vi "Fetch the IO Controls.vi"(0 "VI Path":path, 11 "error in (no error)":errorcluster) -> (4 "IO Controls[]":string[](array[string]), 15 "error out":errorcluster)   [LabVIEW 2021, in "Converter.lvlib"]
uses:
  Converter.lvlib
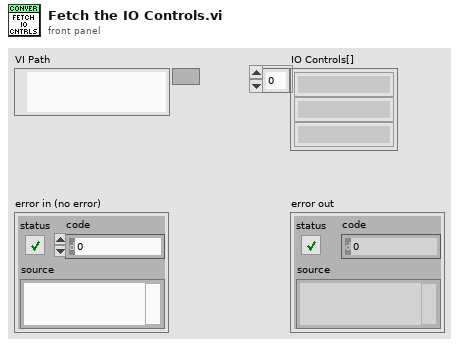
[diagram p1: front panel]
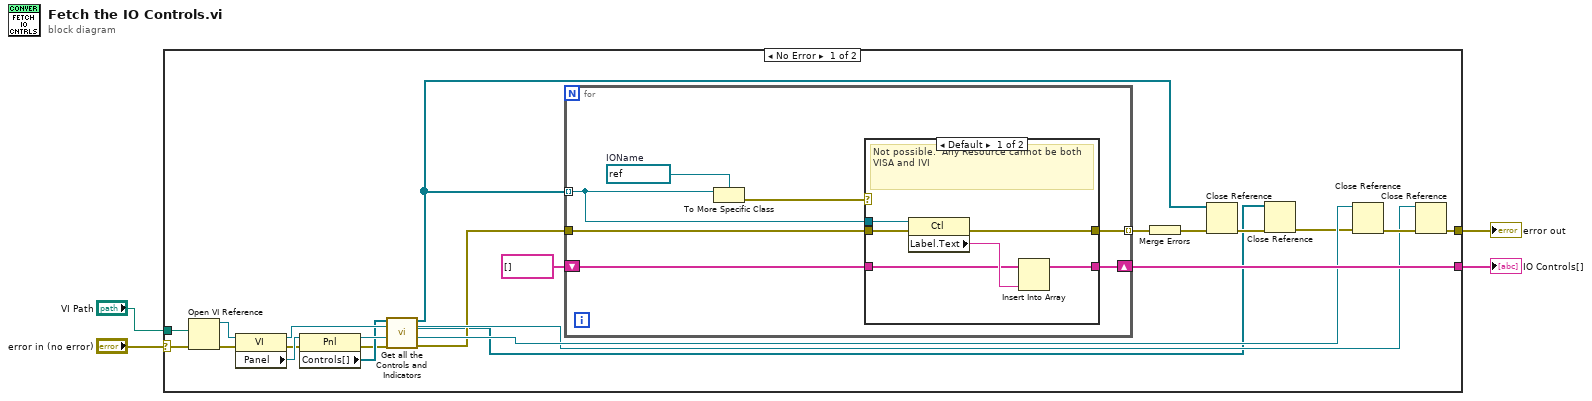
[diagram p0: block diagram]
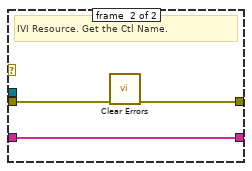
[diagram p2: hidden frame]
diagram:
  n1 = case shown="No Error" "error in (no error)" {
    selector: "error in (no error)" -> [w14 w42]
    tunnel: [w18 _] -> w4
    tunnel: [w13 w42] -> w2
    tunnel: "VI Path" -> [w12 _]
    frame No Error {
      n2 = Open VI Reference(vi path=w12, error in (no error)=w14) -> (vi reference=w25:refnum<vi>, error out=w23:errorcluster)  [unwired: 4 in]
      n3 = property class="VI"(reference=w25, error in=w23) -> (reference out=w15:refnum<vi>, error out=w22:errorcluster, "Panel"=w24:refnum<vi>)
      n4 = property class="Pnl"(reference=w24, error in=w22) -> (reference out=w16:refnum<vi>, error out=w9:errorcluster, "Controls[]"=w11:refnum<vi>[])
      n5 = call "Get all the Controls and Indicators.vi"("Controls[]"=w11, "error in (no error)"=w9) -> ("Controls[]"=w8:refnum<vi>[], "Indicators[]"=w5:refnum<vi>[], "error out"=w10:errorcluster)  [unwired: 11 in]
      n6 = for {
        tunnel: w8 -> [w31] mode=indexing
        tunnel: w10 -> [w30]
        tunnel: [w29] -> w21 mode=indexing
        shift-right: [w27] -> w18
        shift-left: string[] [] -> [w28]
        w32 = refnum<vi> refnum  # IOName
        n7 = To More Specific Class(target class=w32, reference=w31) -> (error out=w26:errorcluster)  [unwired: 1 in, 1 out]
        n8 = case shown="Default" w26 {
          tunnel: w31 -> [w36 _]
          tunnel: [w35 w39] -> w29
          tunnel: w30 -> [w37 w41]
          tunnel: w28 -> [w33 w40]
          tunnel: [w34 w40] -> w27
          frame #0 {
            # "Not possible.  Any Resource cannot be both VISA and IVI"
            n9 = property class="Ctl"(reference=w36, error in=w37) -> (error out=w35:errorcluster, "Label.Text"=w38:string)  [unwired: 1 out]
            n10 = Insert Into Array(array=w33, new element=w38) -> (w34:string[])  [unwired: 1 in]
          }
          frame #1 {
            # "IVI Resource. Get the Ctl Name."
            n11 = call <vilib>:"Clear Errors.vi"("error in (no error)"=w41) -> ("error out"=w39:errorcluster)  [unwired: 5 in, 1 out]
          }
        }
      }
      n12 = Merge Errors(w21) -> (w20:errorcluster)
      n13 = Close Reference(reference=w8, error in (no error)=w20) -> (error out=w7:errorcluster)
      n14 = Close Reference(reference=w5, error in (no error)=w7) -> (error out=w6:errorcluster)
      n15 = Close Reference(reference=w16, error in (no error)=w6) -> (error out=w17:errorcluster)
      n16 = Close Reference(reference=w15, error in (no error)=w17) -> (error out=w13:errorcluster)
    }
    frame Error {
    }
  }
  "error out" <- w2
  "IO Controls[]" <- w4
